vi "SLSC Switch Close.vi"(8 "error in":errorcluster, 11 "slsc switch session":T1) -> (0 "error out":errorcluster)   [LabVIEW 2017, in "NI-SWITCH Scripting.lvlib"]
doc: "This VI works around Bug 898224, which is related to the error parameter for NI-SLSC Switch VIs incorrectly being marked as const. This particularly impacts Close, which attempts to pass a \"no error\" parameter to the CLFN, but will instead pass an error if the VI previously returned one.\n\nBy calling this VI instead of SLSC Switch.lvlib:Close.vi, we can clear errors prior to them reaching the affected call site.\n\nThis helper can be removed when Bug 898224 is fixed in the minimum supported version of NI-SLSC Switch."
uses:
  NI-SWITCH Scripting.lvlib
  <vilib>/userdefined/High Color/SLSC_Switch/nislscslSession.ctl
  <vilib>/SLSC_Switch/SLSC Switch.lvlib
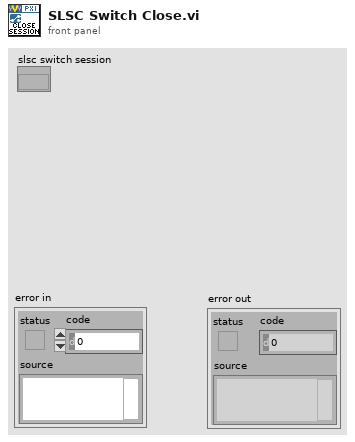
[diagram p1: front panel]
types:
  T1 = typedef "nislscslSession.ctl" = refnum<k20>
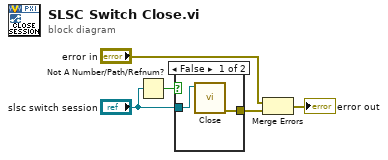
[diagram p0: block diagram]
diagram:
  n1 = Not A Number/Path/Refnum?(number/path/refnum="slsc switch session") -> (NaN/Path/Refnum?=w1:bool)
  n2 = case shown="False" w1 {
    tunnel: [w7 _] -> w4
    tunnel: "slsc switch session" -> [w6 _]
    frame False {
      n3 = call <vilib>:"Close.vi"("session in"=w6) -> ("error out"=w7:errorcluster)  [unwired: 10 in]
    }
    frame True {
    }
  }
  n4 = Merge Errors("error in", w4) -> (→"error out":errorcluster)
